vi "DUAL GAUGE-ConverIntIntEngEng.vi"(0 "String in":string) -> (6 "Integer1 out":u8, 8 "Eng1 out":dbl format="%.3e", 10 "Integer2 out":u8, 15 "Eng2 out":dbl format="%.3e")   [LabVIEW 2017, in "Dual Gauge.lvlib"]
uses:
  <userlib>/Dual Gauge/Dual Gauge.lvlib
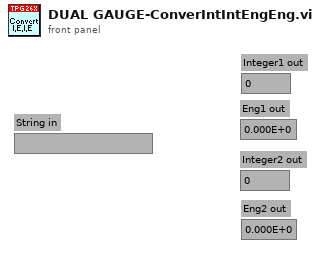
[diagram p1: front panel]
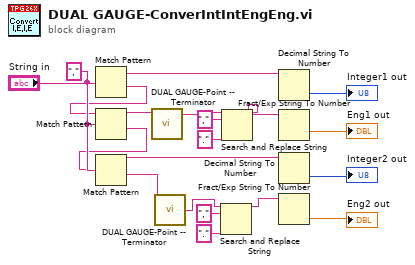
[diagram p0: block diagram]
diagram:
  w16 = "," ("regular expression")
  n1 = Match Pattern(string="String in", regular expression=w16) -> (before substring=w13:string, after substring=w14:string)  [unwired: 1 in, 2 out]
  n2 = Match Pattern(string=w14, regular expression=w16) -> (before substring=w17:string, after substring=w15:string)  [unwired: 1 in, 2 out]
  n3 = Match Pattern(string=w15, regular expression=w16) -> (before substring=w11:string, after substring=w10:string)  [unwired: 1 in, 2 out]
  n4 = call <userlib>:"DUAL GAUGE-Point -- Terminator.vi"("Eingangstring"=w17) -> ("Ausgangstring"=w8:string)
  n5 = call <userlib>:"DUAL GAUGE-Point -- Terminator.vi"("Eingangstring"=w10) -> ("Ausgangstring"=w2:string)
  n6 = Search and Replace String(input string=w2, search string=",", replace string="." ("replace string (\"\")")) -> (result string=w1:string)  [unwired: 5 in, 3 out]
  n7 = Search and Replace String(input string=w8, search string=",", replace string="." ("replace string (\"\")")) -> (result string=w5:string)  [unwired: 5 in, 3 out]
  n8 = Decimal String To Number(string=w13) -> (number=→"Integer1 out":i32)  [unwired: 2 in, 1 out]
  n9 = Fract/Exp String To Number(string=w5) -> (number=→"Eng1 out":dbl)  [unwired: 3 in, 1 out]
  n10 = Decimal String To Number(string=w11) -> (number=→"Integer2 out":i32)  [unwired: 2 in, 1 out]
  n11 = Fract/Exp String To Number(string=w1) -> (number=→"Eng2 out":dbl)  [unwired: 3 in, 1 out]
